vi "Fail If.vi"(7 "Description":string, 8 "error in (no error)":errorcluster, 9 "Message":string, 10 "Fail?":bool, 11 "LUnit Test Case In":refnum<class "LUnit Test Case.lvclass">) -> (0 "error out":errorcluster, 3 "LUnit Test Case Out":refnum<class "LUnit Test Case.lvclass">)   [LabVIEW 2020, in "LUnit Test Case.lvclass"]
doc: "Generates a fail result for the calling test method if the conditional input is true. A description and message may be provided."
uses:
  LUnit Test Case.lvclass
  Result/Type.ctl
  LUnit Test Case.lvclass/LUnit Test Case.ctl
  Private/Run In UI.vi
  <vilib>/Utility/error.llb/Clear Errors.vi
  Result/Result.lvlib
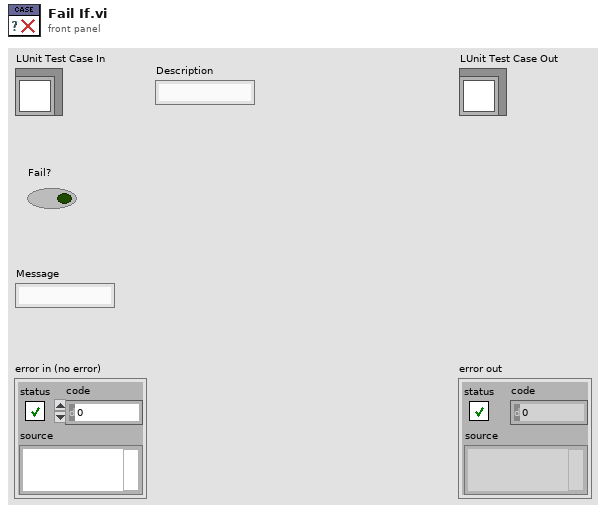
[diagram p1: front panel]
types:
  T1 = typedef "Result.lvlib/Type.ctl" = enum16{"Test Case", "Test Suite", "Test Run", "Pass", "Fail", "Skip", "Pass if", "Fail if", "Pass if Error", "Fail if Error", "Pass if Equal", "Fail if Equal"}
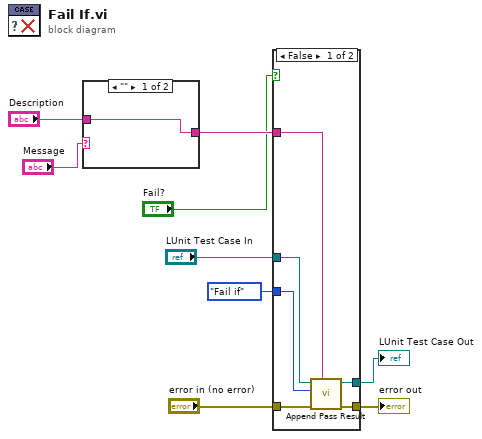
[diagram p0: block diagram]
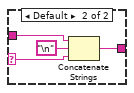
[diagram p2: hidden frame]
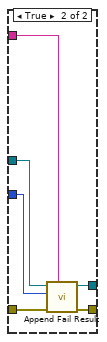
[diagram p3: hidden frame]
diagram:
  n1 = case shown="\"\"" "Message" {
    selector: "Message" -> [_ w12]
    tunnel: "Description" -> [w10 w14]
    tunnel: [w10 w13] -> w3
    frame "" {
    }
    frame Default {
      n2 = Concatenate Strings(w14, "\n", w12) -> (w13:string)
    }
  }
  n3 = case shown="False" "Fail?" {
    tunnel: [w20 w25] -> w9
    tunnel: [w17 w24] -> w7
    tunnel: w3 -> [w18 w23]
    tunnel: "LUnit Test Case In" -> [w19 w26]
    tunnel: "error in (no error)" -> [w16 w22]
    tunnel: Type."Fail if" ("Result Type") -> [w15 w21]
    frame False {
      n4 = call "Append Pass Result.vi"("Description"=w18, "error in (no error)"=w16, "Result Type"=w15, "LUnit Test Case In"=w19) -> ("error out"=w17:errorcluster, "LUnit Test Case Out"=w20:refnum<class "LUnit Test Case.lvclass">)  [unwired: 6 in]
    }
    frame True {
      n5 = call "Append Fail Result.vi"("Description"=w23, "error in (no error)"=w22, "Result Type"=w21, "LUnit Test Case In"=w26) -> ("error out"=w24:errorcluster, "LUnit Test Case Out"=w25:refnum<class "LUnit Test Case.lvclass">)  [unwired: 6 in]
    }
  }
  "error out" <- w7
  "LUnit Test Case Out" <- w9
